vi "List Items On FP Menu.vi"(9 "Item Groups In":T1, 11 "Menu Reference":refnum<k9>) -> ()   [LabVIEW 2024, in "Front Panel Menu.lvclass"]
uses:
  Front Panel Menu.lvclass
  Type Def/Menu Item Group.ctl
  Type Def/Menu Item.ctl
  Type Def/Item Forming Unit.ctl
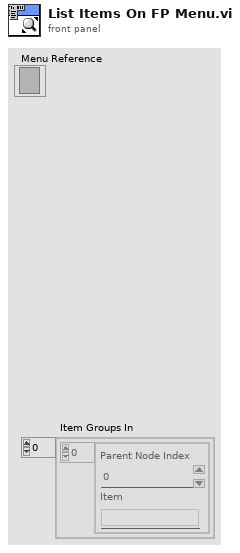
[diagram p1: front panel]
types:
  T1 = typedef "Menu Item Group.ctl" = cluster{"Array":T2[]}[]
  T2 = typedef "Menu Item.ctl" = cluster{"Parent Node Index":i32, "Item":string}
  T3 = typedef "Item Forming Unit.ctl" = cluster{"Parent Tag":string, "Names":string[]}
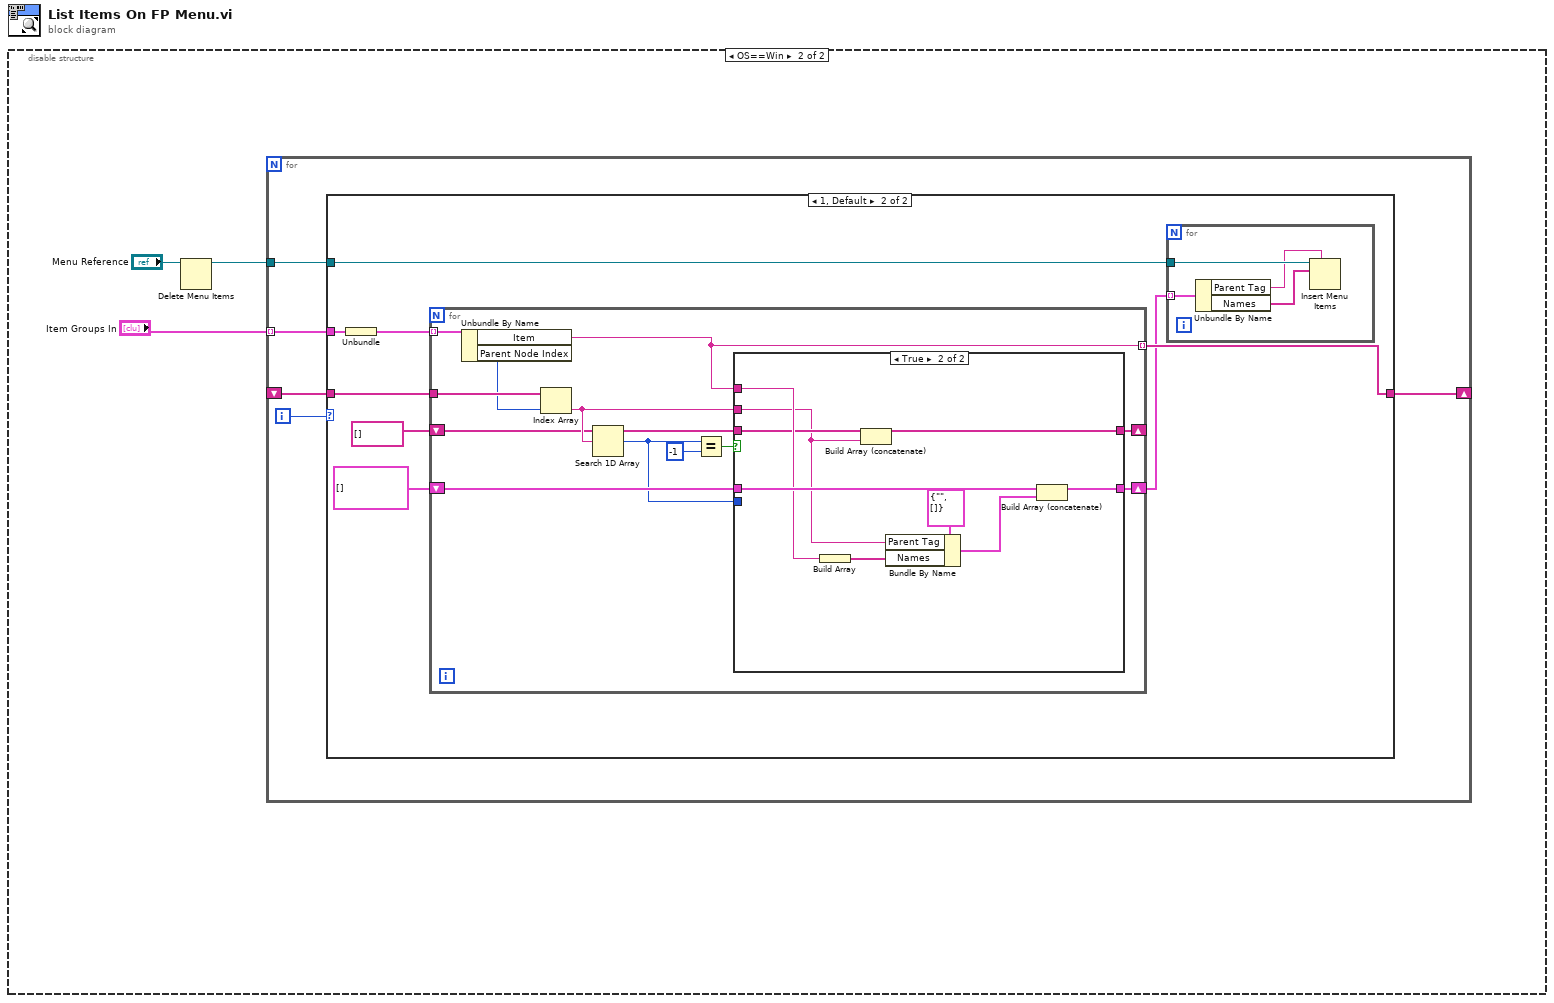
[diagram p0: block diagram]
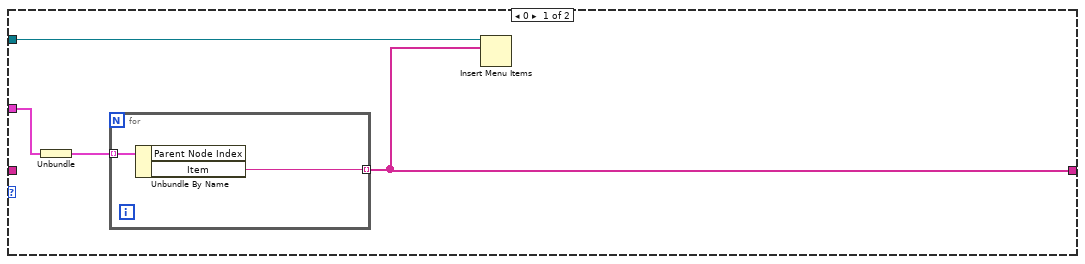
[diagram p3: hidden frame]
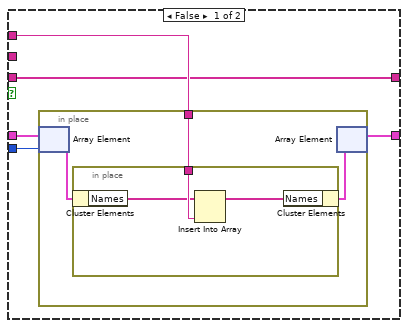
[diagram p4: hidden frame]
diagram:
  n1 = disable-structure shown="OS==Win" {
    frame condition #0 {
    }
    frame condition #1 (active) {
      n2 = Delete Menu Items(9:"Menu Reference") -> (3:w1:refnum<k9>)  [unwired: 3 in, 1 out]
      n3 = for {
        tunnel: "Item Groups In" -> [w6] mode=indexing
        tunnel: w1 -> [w8]
        shift-right: [w5] -> _
        shift-left: _ -> [w4]
        i -> [w7]
        n4 = case shown="1, Default" w7 {
          tunnel: w8 -> [w10 w22]
          tunnel: w6 -> [w12 w20]
          tunnel: [w9 w18] -> w5
          tunnel: w4 -> [_ w19]
          frame 0 {
            n5 = Unbundle(w12) -> ("Array"=w11:T2[])
            n6 = for {
              tunnel: w11 -> [w14] mode=indexing
              tunnel: [w13] -> w9 mode=indexing
              n7 = Unbundle By Name(w14) -> ("Item"=w13:string)  [unwired: 1 out]
            }
            n8 = Insert Menu Items(8:w9, 9:w10) -> ()  [unwired: 4 in, 3 out]
          }
          frame 1, Default {
            n9 = Unbundle(w20) -> ("Array"=w21:T2[])
            n10 = for {
              tunnel: w21 -> [w38] mode=indexing
              tunnel: w19 -> [w37]
              tunnel: [w27] -> w18 mode=indexing
              shift-right: [w35] -> _
              shift-left: string[] [] -> [w29]
              shift-right: [w33] -> w16
              shift-left: T3[] [] -> [w34]
              n11 = Unbundle By Name(w38) -> ("Item"=w27:string, "Parent Node Index"=w36:i32)
              n12 = Index Array(array=w37, index=w36) -> (element=w32:string)
              n13 = Search 1D Array(1D array=w29, element=w32) -> (index of element=w28:i32)  [unwired: 1 in]
              n14 = Equal?(x=w28, y=-1) -> (x = y?=w30:bool)
              n15 = case shown="True" w30 {
                tunnel: [w42 w52] -> w35
                tunnel: w32 -> [_ w53]
                tunnel: w27 -> [w43 w56]
                tunnel: w34 -> [w41 w58]
                tunnel: [w40 w57] -> w33
                tunnel: w29 -> [w42 w54]
                tunnel: w28 -> [w39 _]
                frame False {
                  n16 = in-place {
                    in-place-border: w43 -> [w46]
                    n17 = in-place-array #1(w41, w39) -> (w45:T3)
                    n18 = in-place {
                      in-place-border: w46 -> [w49]
                      n19 = in-place-cluster #2(w45) -> ("Names"=w48:string[])
                      n20 = Insert Into Array(array=w48, new element=w49) -> (w47:string[])  [unwired: 1 in]
                      n21 = in-place-cluster #2("Names"=w47) -> (w44:T3)
                    }
                    n22 = in-place-array #1(w44) -> (w40:T3[])  [unwired: 1 out]
                  }
                }
                frame True {
                  n23 = Build Array(w56) -> (w55:string[])
                  n24 = Build Array (concatenate)(w54, w53) -> (w52:string[])
                  n25 = Bundle By Name(cluster=T3 {"Parent Tag"="", "Names"=[]} ("Item Forming Unit"), "Parent Tag"=w53, "Names"=w55) -> (w51:T3)
                  n26 = Build Array (concatenate)(w58, w51) -> (w57:T3[])
                }
              }
            }
            n27 = for {
              tunnel: w22 -> [w26]
              tunnel: w16 -> [w25] mode=indexing
              n28 = Unbundle By Name(w25) -> ("Parent Tag"=w24:string, "Names"=w23:string[])
              n29 = Insert Menu Items(5:w24, 8:w23, 9:w26) -> ()  [unwired: 3 in, 3 out]
            }
          }
        }
      }
    }
  }
